vi "Coin Flip Start.vi"(8 "error in (no error)":errorcluster, 11 "Reversi in":refnum<class "Reversi.lvclass">) -> (0 "error out":errorcluster, 3 "Reversi out":refnum<class "Reversi.lvclass">)   [LabVIEW 2020, in "Reversi.lvlib" / "Reversi.lvclass"]
uses:
  Reversi.lvclass
  Turn Enum.ctl
  <vilib>/numeric/Random Number (Range) I64.vi
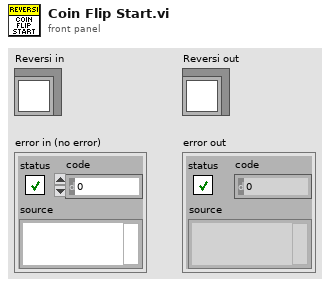
[diagram p1: front panel]
types:
  T1 = typedef "Reversi.lvlib/Reversi.lvclass/Turn Enum.ctl" = enum16{"Black", "White"}
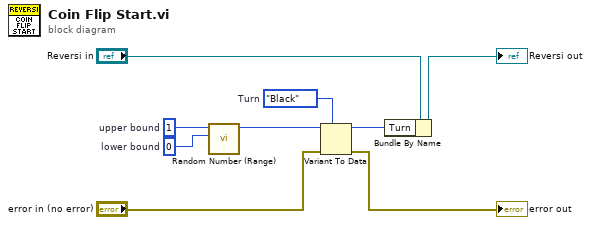
[diagram p0: block diagram]
diagram:
  w4 = Turn_Enum."Black"  # Turn
  w8 = i64 1  # upper bound
  w9 = i64 0  # lower bound
  n1 = call-poly <vilib>:"Random Number (Range).vi"("lower bound (-100)"=w9, "upper bound (100)"=w8) -> ("number"=w5:i64)  [unwired: 9 in]
  n2 = Variant To Data(error in="error in (no error)", type=w4, Variant=w5) -> (data=w3:T1, error out=→"error out":errorcluster)
  n3 = Bundle By Name(cluster="Reversi in", "Turn"=w3) -> (→"Reversi out":refnum<class "Reversi.lvclass">)
